vi "StellarNet Write Spectrometer Coeffs to XML, ext precision.vi"(8 "error in (no error)":errorcluster, 10 "Multi Channel Coefficients & WLs":T1(array[cluster])=[{"Coefficients"=[0.718, 0.00062, 200.0, 0.0], "Wavelengths"=array[2051 elements]}] {"Coefficients" format="%_15g"}, 11 "XML File Path":path=path "C:/program files/StellarNet/SpectraWiz/StellarNet Spectrometer Coefficients.xml") -> (0 "error out":errorcluster)   [LabVIEW 2023]
uses:
  <vilib>/Utility/xml.llb/Write to XML File(string).vi
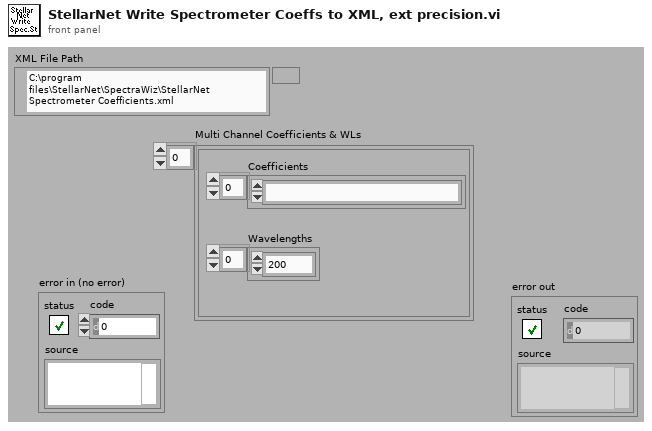
[diagram p1: front panel]
types:
  T1 = cluster{"Coefficients":ext[], "Wavelengths":dbl[]}[]
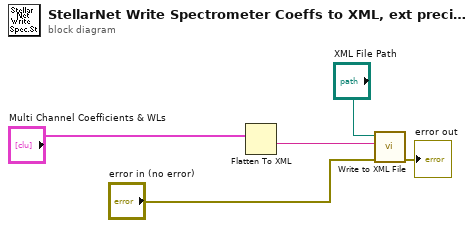
[diagram p0: block diagram]
diagram:
  n1 = Flatten To XML(6:"Multi Channel Coefficients & WLs") -> (2:w5:string)
  n2 = call-poly <vilib>:"Write to XML File.vi"("error in (no error)"="error in (no error)", "XML Input"=w5, "XML File Path"="XML File Path") -> ("error out"=→"error out":errorcluster)  [unwired: 6 in, 2 out]
